vi "Destroy.vi"(8 "error in (no error)":errorcluster, 11 "XRay Table in":refnum<class "XRay Table.lvclass">) -> (0 "error out":errorcluster, 3 "XRay Table out":refnum<class "XRay Table.lvclass">)   [LabVIEW 2026, in "XRay Table.lvclass"]
uses:
  XRay Table.lvclass
  XRay Table.lvclass/XRay Table.ctl
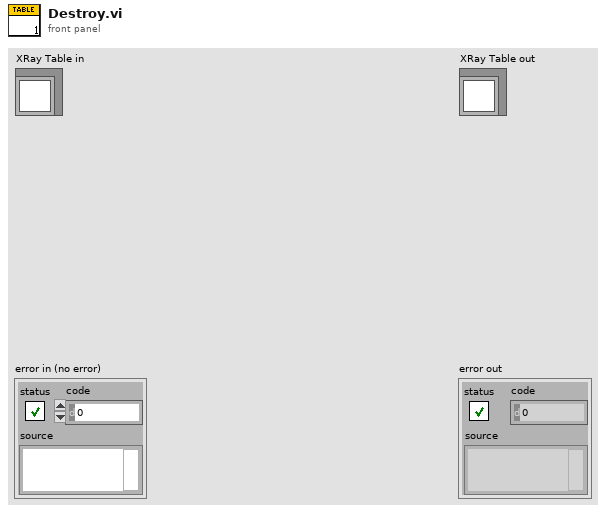
[diagram p1: front panel]
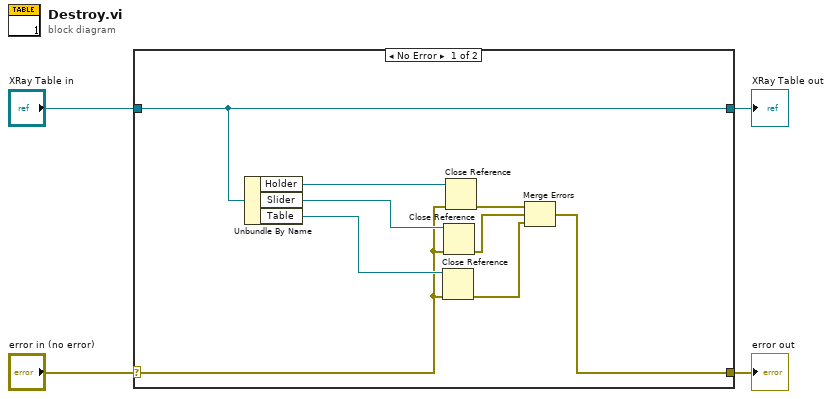
[diagram p0: block diagram]
diagram:
  n1 = case shown="No Error" "error in (no error)" {
    selector: "error in (no error)" -> [w9 w15]
    tunnel: [w5 w15] -> w3
    tunnel: [w13 w14] -> w1
    tunnel: "XRay Table in" -> [w13 w14]
    frame No Error {
      n2 = Unbundle By Name(w13) -> ("Holder"=w12:refnum<vi>, "Slider"=w11:refnum<vi>, "Table"=w10:refnum<vi>)
      n3 = Close Reference(reference=w10, error in (no error)=w9) -> (error out=w6:errorcluster)
      n4 = Close Reference(reference=w11, error in (no error)=w9) -> (error out=w7:errorcluster)
      n5 = Close Reference(reference=w12, error in (no error)=w9) -> (error out=w8:errorcluster)
      n6 = Merge Errors(w8, w7, w6) -> (w5:errorcluster)
    }
    frame Error {
    }
  }
  "error out" <- w3
  "XRay Table out" <- w1
